vi "Agilent 532XX Series Acquire Measurement Statistics.vi"() -> ()   [LabVIEW 2021]
doc: "This example shows how to acquire measurement statistics using the VIs of the driver."
uses:
  <instrlib>/Agilent 532XX Series/Public/Configure/Measurement/Configure Measurement (Frequency).vi
  <instrlib>/Agilent 532XX Series/Public/Data/Read Measurement (Statistics).vi
  <instrlib>/Agilent 532XX Series/Agilent 532XX Series.lvlib
panel:
  in  "Number of Measurement (10)":u32=10
  out "Maximum":dbl format="%#_12g"
  out "Minimum":dbl format="%#_12g"
  out "Standard Deviation":dbl
  out "Mean":dbl format="%#_12g"
  in  "Timeout (10000 ms)":u32=10000
  in  "VISA resource name":refnum<visa-resource-name>
  # "(c) 2010-2015 National Instruments.  ALL RIGHTS RESERVED."
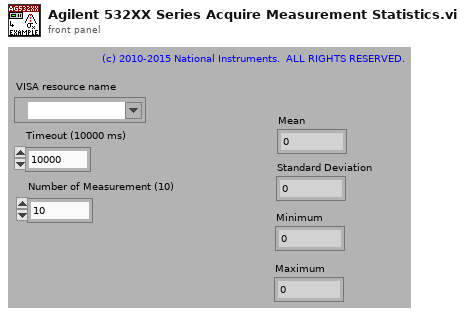
[diagram p1: front panel]
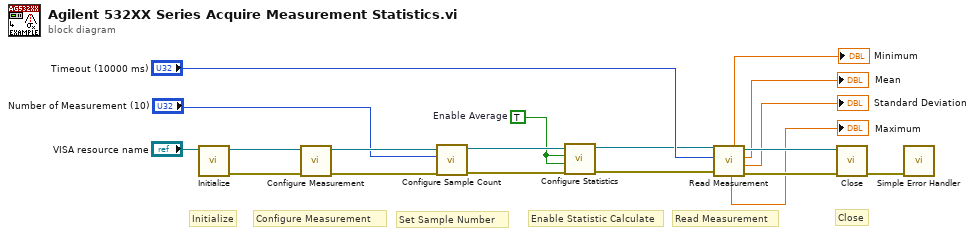
[diagram p0: block diagram]
diagram:
  w2 = TRUE  # Enable Average
  # "Enable Statistic Calculate"
  # "Set Sample Number"
  # "Close"
  # "Read Measurement"
  # "Initialize"
  # "Configure Measurement"
  n1 = call <instrlib>:"Initialize.vi"("VISA resource name"="VISA resource name") -> ("error out"=w16:errorcluster, "VISA resource name out"=w17:refnum<visa-resource-name>)  [unwired: 3 in, 6 out]
  n2 = call-poly <instrlib>:"Configure Measurement.vi"("error in (no error)"=w16, "VISA resource name"=w17) -> ("error out"=w8:errorcluster, "VISA resource name out"=w9:refnum<visa-resource-name>)  [unwired: 3 in, 5 out]
  n3 = call <instrlib>:"Configure Sample Count.vi"("error in (no error)"=w8, "Sample Count (1)"="Number of Measurement (10)", "VISA resource name"=w9) -> ("error out"=w5:errorcluster, "VISA resource name out"=w6:refnum<visa-resource-name>)  [unwired: 7 out]
  n4 = call <instrlib>:"Configure Statistics.vi"("error in (no error)"=w5, "Enable Calculate1 (T: Enable)"=w2, "Enable Average (T: Enable)"=w2, "VISA resource name"=w6) -> ("error out"=w3:errorcluster, "VISA resource name out"=w4:refnum<visa-resource-name>)  [unwired: 6 out]
  n5 = call-poly <instrlib>:"Read Measurement.vi"("error in (no error)"=w3, "Timeout (10000 ms)"="Timeout (10000 ms)", "VISA resource name"=w4) -> ("error out"=w14:errorcluster, "Standard Deviation"=→"Standard Deviation":dbl, "Mean"=→"Mean":dbl, "VISA resource name out"=w13:refnum<visa-resource-name>, "Maximum"=→"Maximum":dbl, "Minimum"=→"Minimum":dbl)  [unwired: 3 out]
  n6 = call <instrlib>:"Close.vi"("error in (no error)"=w14, "VISA resource name"=w13) -> ("error out"=w18:errorcluster)  [unwired: 9 out]
  n7 = call <vilib>:"Simple Error Handler.vi"("error in (no error)"=w18) -> ()  [unwired: 1 in, 8 out]
